vi "Main.vi"(8 "error in":errorcluster, 11 "Work Planer in":refnum<class "Work Planer.lvclass">) -> (0 "error out":errorcluster, 3 "Work Planer out":refnum<class "Work Planer.lvclass">)   [LabVIEW 2023, in "Work Planer.lvclass"]
doc: "The <b>Queued Message Handler</b> of the Worker that owns this VI."
uses:
  Work Planer.lvclass
  Initialization Data.ctl
  Response Cases.ctl
  <vilib>/addons/_Workers/Library/Case Label.ctl
  <vilib>/addons/_Workers/Library/Classes/Message/Priority (ALL).ctl
  Work Planer.lvclass/Work Planer.ctl
  rsp_Timeout.ctl
  <vilib>/addons/_Workers/Library/Classes/Message/Message.lvclass
  <vilib>/addons/_Workers/Library/Workers.lvlib
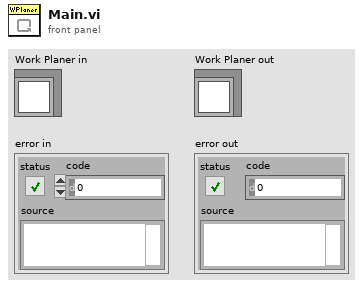
[diagram p1: front panel]
types:
  T1 = typedef "Work Planer.lvclass/Initialization Data.ctl" = cluster{"Response Cases":T2, "Time Precission (100ms)":u32, "Continius? (F)":bool, "Data":variant, "Auxiliary":variant, "Priority (Normal)":T4, "Timeout (1000ms)":u32, "Debugger MSG? (T)":bool}
  T2 = typedef "Work Planer.lvclass/Response Cases.ctl" = cluster{"Timeout":T3}
  T3 = typedef "Workers.lvlib/Case Label.ctl" = string
  T4 = typedef "Workers.lvlib/Message.lvclass/Priority (ALL).ctl" = enum16{"Low", "Normal", "High", "Critical"}
  T5 = typedef "Work Planer.lvclass/rsp_Timeout.ctl" = cluster{"Data":variant, "Auxiliary":variant}
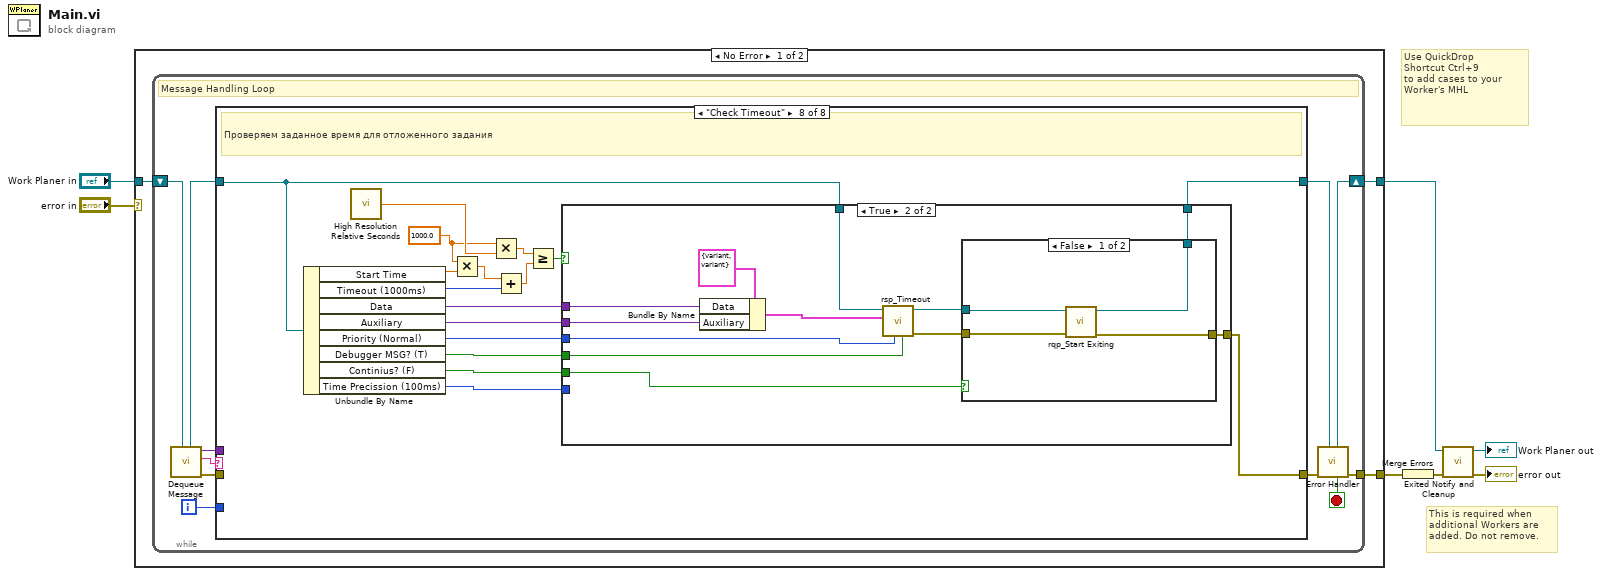
[diagram p0: block diagram]
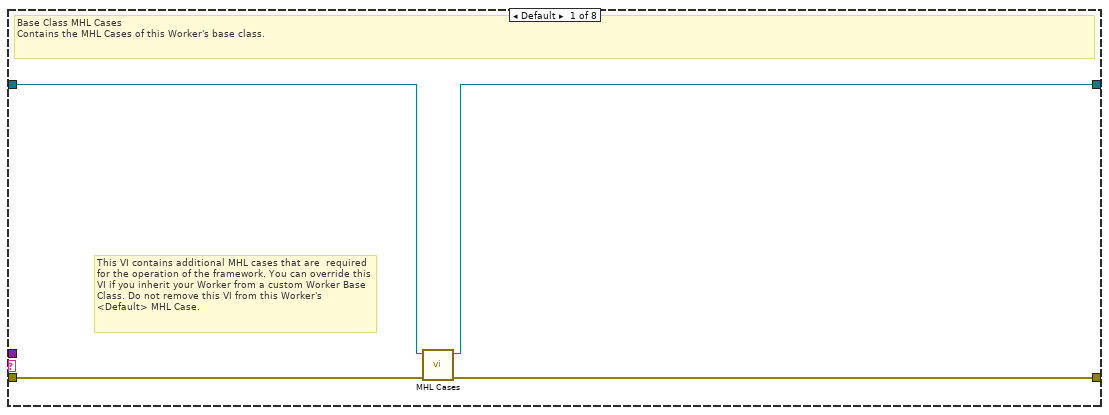
[diagram p2: hidden frame]
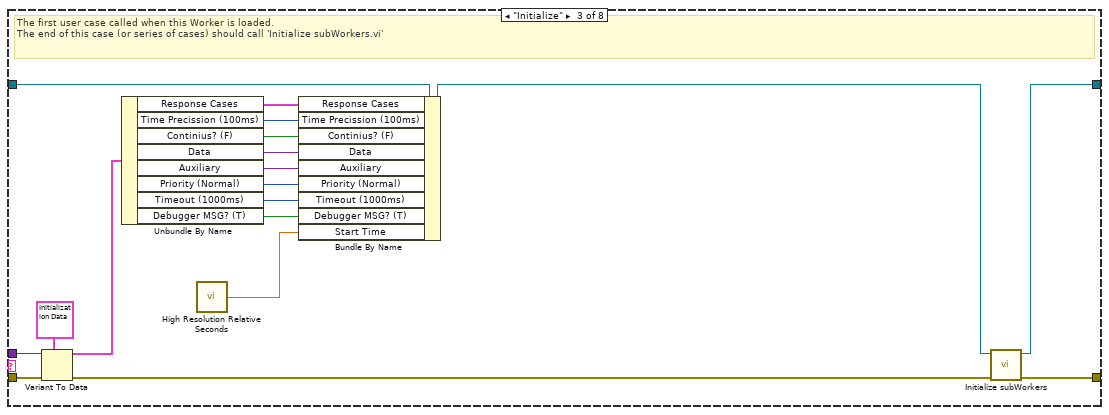
[diagram p4: hidden frame]
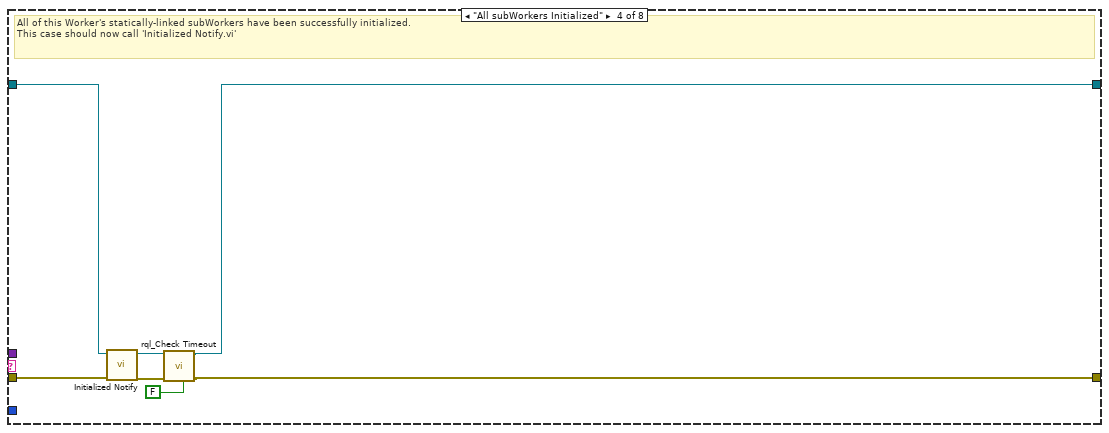
[diagram p5: hidden frame]
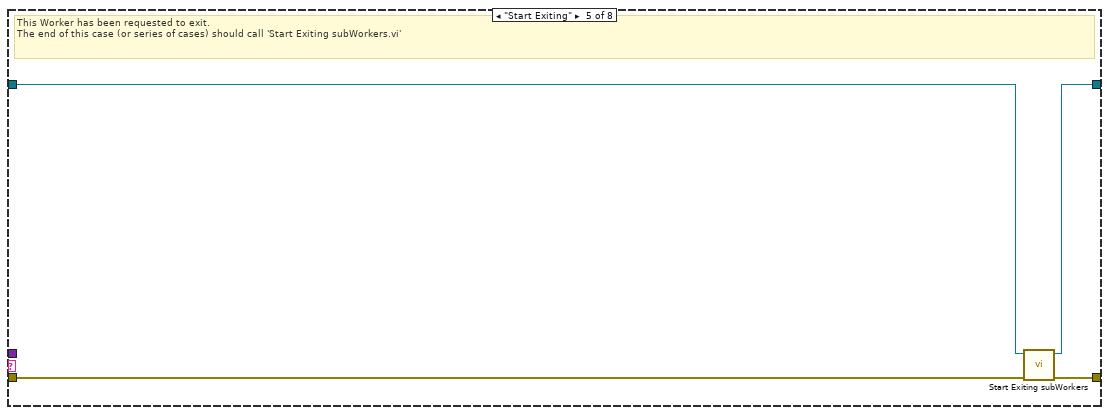
[diagram p6: hidden frame]
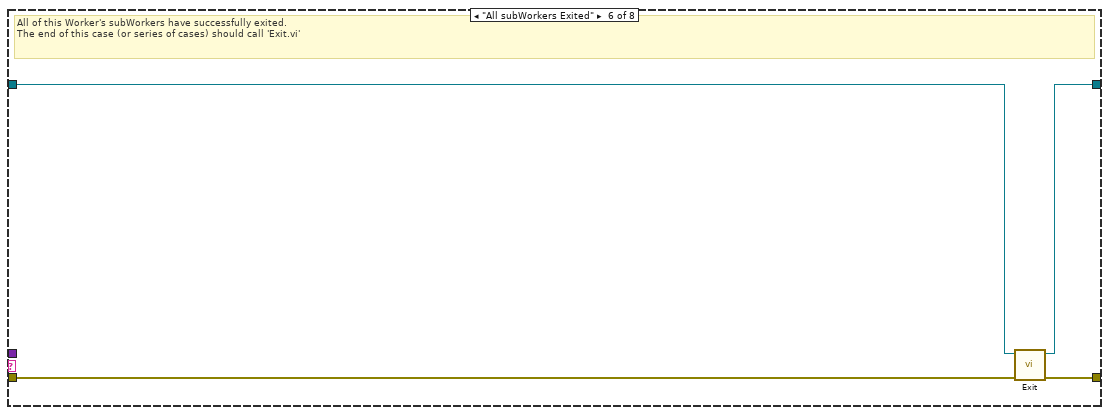
[diagram p7: hidden frame]
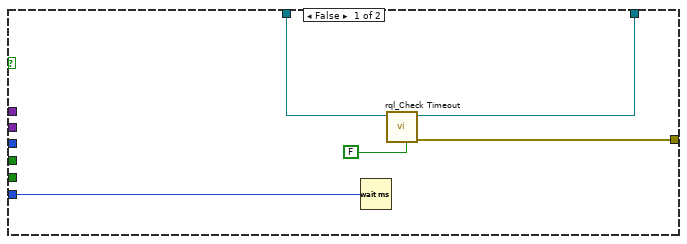
[diagram p9: hidden frame]
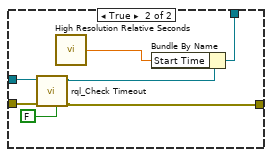
[diagram p10: hidden frame]
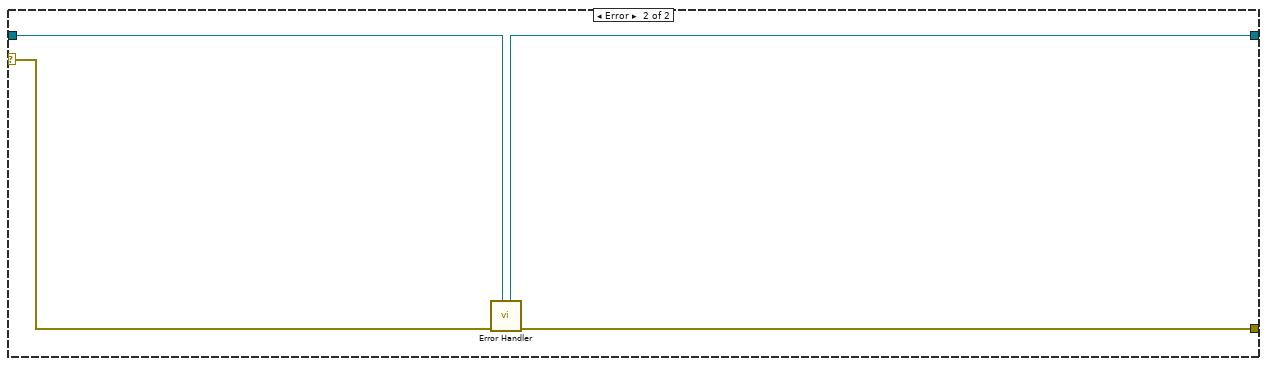
[diagram p11: hidden frame]
diagram:
  # "Use QuickDrop\nShortcut Ctrl+9\nto add cases to your\nWorker's MHL"
  # "This is required when additional Workers are added. Do not remove."
  n1 = case shown="No Error" "error in" {
    tunnel: "Work Planer in" -> [w8 w109]
    tunnel: [w10 w110] -> w6
    tunnel: [w9 w108] -> w7
    selector: "error in" -> [_ w111]
    frame No Error {
      n2 = while {
        shift-right: [w19] -> w9
        shift-left: w8 -> [w21]
        tunnel: [w20] -> w10
        i -> [w12]
        stop <- w13 stop-if-true
        # "Message Handling Loop"
        n3 = call-dynamic "Dequeue Message.vi"("Worker"=w21) -> ("error out"=w18:errorcluster, "Case out"=w14:string, "Data out"=w11:variant, "Worker out"=w16:refnum<class "Work Planer.lvclass">)  [unwired: 6 in, 1 out]
        n4 = case "Worker MHL Case Structure (DO NOT CHANGE LABEL NAME)" shown="\"Check Timeout\"" w14 {
          tunnel: w18 -> [w25 w26 w43 w52 w53 w60 w62 _]
          tunnel: [w24 w26 w45 w47 w56 w59 w62 w63] -> w17
          tunnel: w16 -> [w23 w27 w42 w51 w54 w58 w61 w65]
          tunnel: [w22 w27 w44 w48 w55 w57 w61 w64] -> w15
          tunnel: w12 -> [_ _ _ _ _ _ _ _]
          tunnel: w11 -> [_ _ w40 _ _ _ _ _]
          frame Default {
            # "This VI contains additional MHL cases that are  required for the operation of the framework. You can override this VI if you inherit your Worker from a custom Worker Base Class. Do not remove this VI from this Worker's <Default> MHL Case."
            # "Base Class MHL Cases\nContains the MHL Cases of this Worker's base class."
            n5 = call-dynamic "MHL Cases.vi"("error in"=w25, "Worker in"=w23) -> ("error out"=w24:errorcluster, "Worker out"=w22:refnum<class "Work Planer.lvclass">)  [unwired: 8 in]
          }
          frame "------------ FRAMEWORK CASES -----------" {
            # "Start of Workers Framework Cases"
          }
          frame "Initialize" {
            # "The first user case called when this Worker is loaded.\nThe end of this case (or series of cases) should call 'Initialize subWorkers.vi'"
            n6 = Variant To Data(error in=w43, type=T1 {"Response Cases"={"Timeout"=""}, "Time Precission (100ms)"=100, "Continius? (F)"=FALSE, "Data"=variant, "Auxiliary"=variant, "Priority (Normal)"=enum."Normal", "Timeout (1000ms)"=1000, "Debugger MSG? (T)"=TRUE} ("Cluster"), Variant=w40) -> (data=w38:T1, error out=w41:errorcluster)
            n7 = Unbundle By Name(w38) -> ("Response Cases"=w37:T2, "Time Precission (100ms)"=w35:u32, "Continius? (F)"=w34:bool, "Data"=w33:variant, "Auxiliary"=w32:variant, "Priority (Normal)"=w31:T4, "Timeout (1000ms)"=w30:u32, "Debugger MSG? (T)"=w29:bool)
            n8 = call <vilib>:"High Resolution Relative Seconds.vi"() -> ("relative seconds"=w28:dbl)
            n9 = Bundle By Name(cluster=w42, "Response Cases"=w37, "Time Precission (100ms)"=w35, "Continius? (F)"=w34, "Data"=w33, "Auxiliary"=w32, "Priority (Normal)"=w31, "Timeout (1000ms)"=w30, "Debugger MSG? (T)"=w29, "Start Time"=w28) -> (w39:refnum<class "Work Planer.lvclass">)
            n10 = call-dynamic "Initialize subWorkers.vi"("error in"=w41, "Worker"=w39) -> ("error out"=w45:errorcluster, "dup Worker out"=w44:refnum<class "Work Planer.lvclass">)  [unwired: 8 in]
          }
          frame "All subWorkers Initialized" {
            # "All of this Worker's statically-linked subWorkers have been successfully initialized.\nThis case should now call 'Initialized Notify.vi'"
            n11 = call-dynamic "Initialized Notify.vi"("error in"=w52, "Worker"=w51) -> ("error out"=w50:errorcluster, "dup Worker out"=w49:refnum<class "Work Planer.lvclass">)  [unwired: 8 in]
            n12 = call "rql_Check Timeout.vi"("Show in Debugger?"=FALSE, "error in"=w50, "Work Planer in"=w49) -> ("error out"=w47:errorcluster, "dup Work Planer out"=w48:refnum<class "Work Planer.lvclass">)  [unwired: 7 in]
          }
          frame "Start Exiting" {
            # "This Worker has been requested to exit. \nThe end of this case (or series of cases) should call 'Start Exiting subWorkers.vi'"
            n13 = call-dynamic "Start Exiting subWorkers.vi"("error_in"=w53, "Worker"=w54) -> ("error out"=w56:errorcluster, "dup Worker out"=w55:refnum<class "Work Planer.lvclass">)  [unwired: 8 in]
          }
          frame "All subWorkers Exited" {
            # "All of this Worker's subWorkers have successfully exited. \nThe end of this case (or series of cases) should call 'Exit.vi'"
            n14 = call-dynamic "Exit.vi"("error_in"=w60, "Worker"=w58) -> ("error out"=w59:errorcluster, "dup Worker out"=w57:refnum<class "Work Planer.lvclass">)  [unwired: 8 in]
          }
          frame "------------- LOCAL API CASES -------------" {
            # "Start of Workers Local API Cases"
          }
          frame "Check Timeout" {
            w66 = 1000.0 ("x")
            # "Проверяем заданное время для отложенного задания"
            n15 = Unbundle By Name(w65) -> ("Start Time"=w76:dbl, "Timeout (1000ms)"=w77:u32, "Data"=w74:variant, "Auxiliary"=w73:variant, "Priority (Normal)"=w72:T4, "Debugger MSG? (T)"=w71:bool, "Continius? (F)"=w70:bool, "Time Precission (100ms)"=w69:u32)
            n16 = call <vilib>:"High Resolution Relative Seconds.vi"() -> ("relative seconds"=w79:dbl)
            n17 = Multiply(x=w66, y=w76) -> (x*y=w68:dbl)
            n18 = Multiply(x=w66, y=w79) -> (x*y=w67:dbl)
            n19 = Add(x=w68, y=w77) -> (x+y=w78:dbl)
            n20 = Greater Or Equal?(x=w67, y=w78) -> (x >= y?=w75:bool)
            n21 = case shown="True" w75 {
              tunnel: w65 -> [w83 w89]
              tunnel: [w82 w95] -> w64
              tunnel: w74 -> [_ w86]
              tunnel: w73 -> [_ w85]
              tunnel: w72 -> [_ w90]
              tunnel: w71 -> [_ w91]
              tunnel: w70 -> [_ w96]
              tunnel: [w81 w94] -> w63
              tunnel: w69 -> [w84 _]
              frame False {
                n22 = Wait (ms)(milliseconds to wait=w84) -> ()  [unwired: 1 out]
                n23 = call "rql_Check Timeout.vi"("Show in Debugger?"=FALSE, "Work Planer in"=w83) -> ("error out"=w81:errorcluster, "dup Work Planer out"=w82:refnum<class "Work Planer.lvclass">)  [unwired: 8 in]
              }
              frame True {
                n24 = Bundle By Name(cluster=T5 {"Data"=variant(string ""), "Auxiliary"=variant} ("Data in"), "Data"=w86, "Auxiliary"=w85) -> (w87:T5)
                n25 = call "rsp_Timeout.vi"("Show in Debugger?"=w91, "Message Priority"=w90, "Data in"=w87, "Work Planer in"=w89) -> ("error out"=w93:errorcluster, "dup Work Planer out"=w92:refnum<class "Work Planer.lvclass">)  [unwired: 6 in]
                n26 = case shown="False" w96 {
                  tunnel: [w99 w106] -> w95
                  tunnel: [w100 w104] -> w94
                  tunnel: w93 -> [w97 w102]
                  tunnel: w92 -> [w98 w101]
                  frame False {
                    n27 = call "rqp_Start Exiting.vi"("error in"=w97, "Work Planer in"=w98) -> ("error out"=w100:errorcluster, "dup Work Planer out"=w99:refnum<class "Work Planer.lvclass">)  [unwired: 7 in, 1 out]
                  }
                  frame True {
                    n28 = call "rql_Check Timeout.vi"("Show in Debugger?"=FALSE, "error in"=w102, "Work Planer in"=w101) -> ("error out"=w104:errorcluster, "dup Work Planer out"=w103:refnum<class "Work Planer.lvclass">)  [unwired: 7 in]
                    n29 = call <vilib>:"High Resolution Relative Seconds.vi"() -> ("relative seconds"=w107:dbl)
                    n30 = Bundle By Name(cluster=w103, "Start Time"=w107) -> (w106:refnum<class "Work Planer.lvclass">)
                  }
                }
              }
            }
          }
        }
        n31 = call-dynamic "Error Handler.vi"("Worker"=w15, "error_in"=w17) -> ("error out"=w20:errorcluster, "Stop Loop"=w13:bool, "Worker out"=w19:refnum<class "Work Planer.lvclass">)  [unwired: 7 in]
      }
    }
    frame Error {
      n32 = call-dynamic "Error Handler.vi"("Worker"=w109, "error_in"=w111) -> ("error out"=w110:errorcluster, "Worker out"=w108:refnum<class "Work Planer.lvclass">)  [unwired: 7 in, 1 out]
    }
  }
  n33 = Merge Errors(w6) -> (w3:errorcluster)
  n34 = call-dynamic "Exited Notify and Cleanup.vi"("error_in"=w3, "Worker"=w7) -> ("error out"=→"error out":errorcluster, "dup Worker out"=→"Work Planer out":refnum<class "Work Planer.lvclass">)  [unwired: 8 in]
